vi "Eraser.vi"(8 "error in (no error)":errorcluster, 9 "point(x,y)":cluster{"x":i16, "y":i16}, 10 "Radio Buttons":T8=enum."Ellipse", 11 "Data in":T1={"Class"={"Ants"=refnum, "Layer"=refnum, "Templates"=refnum, "Icon"=refnum, "Glyph"=refnum, "Settings"=refnum, "Tools"=refnum}, "Ref"={"Add Layer"=refnum, "Remove Layer"=refnum, "Line Text"=[], "Body Text Spec"=refnum, "DNL_Font"=refnum, "glyph path str"=refnum, "templates path str"=refnum, "Arrow Up"=refnum, "Arrow Down"=refnum, "IE VI Ref"=refnum, "Glyphs tree"=refnum, "Templates tree"=refnum, "Layer Icon Text"=refnum, "Layer Template"=refnum, "Body Text"=refnum, "Search Templates"=refnum, "TextMarker"=refnum, "Tab Control"=refnum, "Search Glyphs"=refnum, "Line Color"=refnum, "DNL_Glyphs []"=refnum, "Fill Color"=refnum, "Tools"=refnum, "Icon"=refnum, "Preview"=refnum, "Ants"=refnum, "Terminals"=refnum, "menu reference"=refnum, "LayerNames"=[], "GlyphLoadAnimation"=refnum, "TemplateLoadAnimation"=refnum, "refreshGlyphs"=refnum, "refreshTemplates"=refnum}, "Support"={"AntsRect"={"left"=0, "top"=0, "right"=0, "bottom"=0}, "Mouse Move Coords"={"Horizontal"=0, "Vertical"=0}, "Mouse Down Coords"={"Horizontal"=0, "Vertical"=0}, "Temp Coord"={"Horizontal"=0, "Vertical"=0}, "Action"=enum."Default", "Edge Color"=4914962, "Fill Color"=16860, "Mouse Down?"=FALSE, "Draft Mode?"=FALSE, "Temp Icon"=bytes[3102], "CTRL Pressed"=FALSE, "Move Selection?"=FALSE, "AntsRect Orig"={"left"=0, "top"=0, "right"=0, "bottom"=0}, "Text"="", "TM Set?"=FALSE, "Mouse inside icon?"=FALSE, "Tool (old value)"=0, "Pencil Move Color"=0, "Swap Colors?"=FALSE, "Shift pressed?"=FALSE}}) -> (0 "error out":errorcluster, 3 "Data out":T1={"Class"={"Ants"=refnum, "Layer"=refnum, "Templates"=refnum, "Icon"=refnum, "Glyph"=refnum, "Settings"=refnum, "Tools"=refnum}, "Ref"={"Add Layer"=refnum, "Remove Layer"=refnum, "Line Text"=[], "Body Text Spec"=refnum, "DNL_Font"=refnum, "glyph path str"=refnum, "templates path str"=refnum, "Arrow Up"=refnum, "Arrow Down"=refnum, "IE VI Ref"=refnum, "Glyphs tree"=refnum, "Templates tree"=refnum, "Layer Icon Text"=refnum, "Layer Template"=refnum, "Body Text"=refnum, "Search Templates"=refnum, "TextMarker"=refnum, "Tab Control"=refnum, "Search Glyphs"=refnum, "Line Color"=refnum, "DNL_Glyphs []"=refnum, "Fill Color"=refnum, "Tools"=refnum, "Icon"=refnum, "Preview"=refnum, "Ants"=refnum, "Terminals"=refnum, "menu reference"=refnum, "LayerNames"=[], "GlyphLoadAnimation"=refnum, "TemplateLoadAnimation"=refnum, "refreshGlyphs"=refnum, "refreshTemplates"=refnum}, "Support"={"AntsRect"={"left"=0, "top"=0, "right"=0, "bottom"=0}, "Mouse Move Coords"={"Horizontal"=0, "Vertical"=0}, "Mouse Down Coords"={"Horizontal"=0, "Vertical"=0}, "Temp Coord"={"Horizontal"=0, "Vertical"=0}, "Action"=enum."Default", "Edge Color"=4914962, "Fill Color"=16860, "Mouse Down?"=FALSE, "Draft Mode?"=FALSE, "Temp Icon"=bytes[3102], "CTRL Pressed"=FALSE, "Move Selection?"=FALSE, "AntsRect Orig"={"left"=0, "top"=0, "right"=0, "bottom"=0}, "Text"="", "TM Set?"=FALSE, "Mouse inside icon?"=FALSE, "Tool (old value)"=0, "Pencil Move Color"=0, "Swap Colors?"=FALSE, "Shift pressed?"=FALSE}})   [LabVIEW 2021, in "Tools Paint.lvclass"]
uses:
  <resource>/plugins/NIIconEditor/Class/Tools/Tools Paint.lvclass
  <resource>/plugins/NIIconEditor/Controls/Tools.ctl
  <resource>/plugins/NIIconEditor/Controls/Pen.ctl
  <resource>/plugins/NIIconEditor/Controls/Line.ctl
  <resource>/plugins/NIIconEditor/Controls/Dropper.ctl
  <resource>/plugins/NIIconEditor/Controls/Fill.ctl
  <resource>/plugins/NIIconEditor/Controls/IERect.ctl
  <resource>/plugins/NIIconEditor/Controls/FRect.ctl
  <resource>/plugins/NIIconEditor/Controls/Circle.ctl
  <resource>/plugins/NIIconEditor/Controls/FCircle.ctl
  <resource>/plugins/NIIconEditor/Controls/Rubber.ctl
  <resource>/plugins/NIIconEditor/Controls/Text.ctl
  <resource>/plugins/NIIconEditor/Controls/Selection.ctl
  <resource>/plugins/NIIconEditor/Controls/Move.ctl
  <resource>/plugins/NIIconEditor/Controls/Global Data.ctl
  <resource>/plugins/NIIconEditor/Class/Ants/Ants.lvclass
  <resource>/plugins/NIIconEditor/Class/FakedArray/FakedArray.lvclass
  <vilib>/LabVIEW Icon API/lv_icon/Classes/Icon/Icon.lvclass
  <resource>/plugins/NIIconEditor/Class/Icon Library/Glyph.lvclass
  <resource>/plugins/NIIconEditor/Class/Settings/Settings.lvclass
  <resource>/plugins/NIIconEditor/Controls/IE Classes.ctl
  <resource>/plugins/NIIconEditor/Controls/References Cluster.ctl
  <resource>/plugins/NIIconEditor/Controls/SupportClass.ctl
  <vilib>/Utility/miscctls.llb/LVPoint32TypeDef.ctl
  <resource>/plugins/NIIconEditor/Controls/SupportClass_Action.ctl
  <vilib>/LabVIEW Icon API/lv_icon/Controls/IEColor.ctl
  <vilib>/LabVIEW Icon API/lv_icon/Classes/Icon Framework/Icon Framework.lvclass
  C:/Users/J63553/Projects/_LabVIEW Community/labview-icon-editor/vi.lib/LabVIEW Icon API/lv_icon/Classes/Layer/Layer.lvclass
  <vilib>/LabVIEW Icon API/lv_icon/lv_icon.lvlib
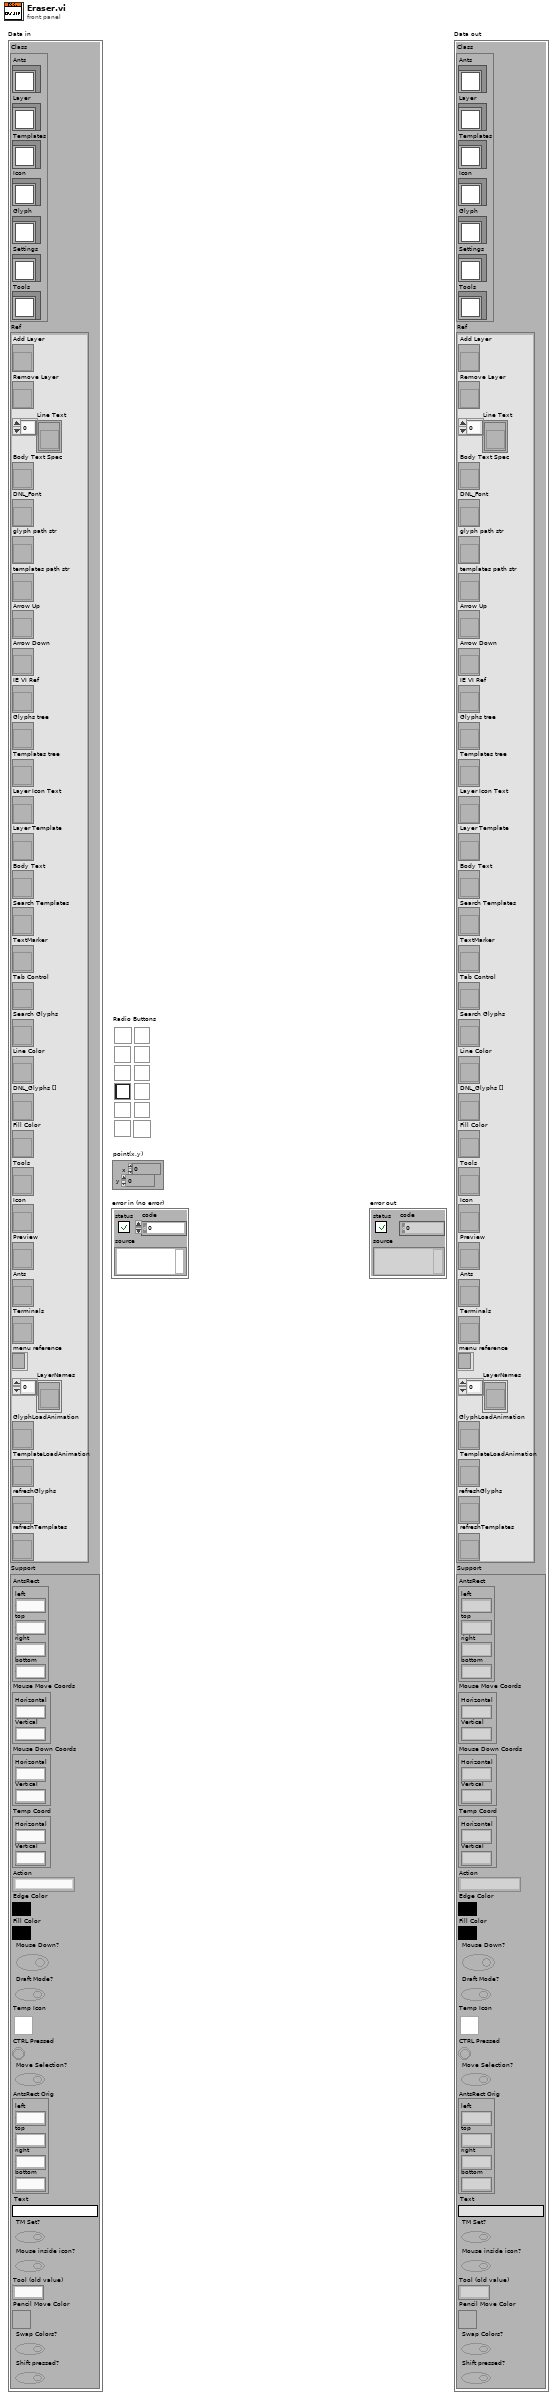
[diagram p1: front panel]
types:
  T1 = typedef "lv_icon.lvlib/Global Data.ctl" = cluster{"Class":T2, "Ref":T3, "Support":T4}
  T2 = typedef "IE Classes.ctl" = cluster{"Ants":refnum<class "Ants.lvclass">, "Layer":refnum<class "FakedArray.lvclass">, "Templates":refnum<class "FakedArray.lvclass">, "Icon":refnum<class "Icon.lvclass">, "Glyph":refnum<class "Glyph.lvclass">, "Settings":refnum<class "Settings.lvclass">, "Tools":refnum<class "Tools Paint.lvclass">}
  T3 = typedef "lv_icon.lvlib/References Cluster.ctl" = cluster{"Add Layer":refnum<vi>, "Remove Layer":refnum<vi>, "Line Text":refnum<vi>[], "Body Text Spec":refnum<vi>, "DNL_Font":refnum<vi>, "glyph path str":refnum<vi>, "templates path str":refnum<vi>, "Arrow Up":refnum<vi>, "Arrow Down":refnum<vi>, "IE VI Ref":refnum<vi>, "Glyphs tree":refnum<vi>, "Templates tree":refnum<vi>, "Layer Icon Text":refnum<vi>, "Layer Template":refnum<vi>, "Body Text":refnum<vi>, "Search Templates":refnum<vi>, "TextMarker":refnum<vi>, "Tab Control":refnum<vi>, "Search Glyphs":refnum<vi>, "Line Color":refnum<vi>, "DNL_Glyphs []":refnum<vi>, "Fill Color":refnum<vi>, "Tools":refnum<vi>, "Icon":refnum<vi>, "Preview":refnum<vi>, "Ants":refnum<vi>, "Terminals":refnum<vi>, "menu reference":refnum<k9>, "LayerNames":refnum<vi>[], "GlyphLoadAnimation":refnum<vi>, "TemplateLoadAnimation":refnum<vi>, "refreshGlyphs":refnum<vi>, "refreshTemplates":refnum<vi>}
  T4 = typedef "SupportClass.ctl" = cluster{"AntsRect":cluster{"left":i16, "top":i16, "right":i16, "bottom":i16}, "Mouse Move Coords":T5, "Mouse Down Coords":T5, "Temp Coord":T5, "Action":T6, "Edge Color":T7, "Fill Color":T7, "Mouse Down?":bool, "Draft Mode?":bool, "Temp Icon":picture, "CTRL Pressed":bool, "Move Selection?":bool, "AntsRect Orig":cluster{"left":i16, "top":i16, "right":i16, "bottom":i16}, "Text":string, "TM Set?":bool, "Mouse inside icon?":bool, "Tool (old value)":u32, "Pencil Move Color":u32, "Swap Colors?":bool, "Shift pressed?":bool}
  T5 = typedef "LVPoint32TypeDef.ctl" = cluster{"Horizontal":i32, "Vertical":i32}
  T6 = typedef "SupportClass_Action.ctl" = enum16{"Default", "Move Selection", "Glyph Library", "Tool"}
  T7 = typedef "IEColor.ctl" = u32
  T8 = typedef "Tools.ctl" = enum32{"Pencil", "Line", "Dropper", "Fill", "Rectangle", "Filled Rectangle", "Ellipse", "Filled Ellipse", "Eraser", "Text", "Select", "Move"}
  T9 = typedef "lv_icon.lvlib/INI Data.ctl" = cluster{"Show Terminals?":bool, "Text":cluster{"Font":T10, "Alignment":T11, "Size":T12}, "3rd party Templates":cluster{"Store 3rd party Templates?":bool, "Folder Name":string}, "Merge user layers on commit":bool, "Body Text":T13, "Fill Color":T7, "Edge Color":T7, "Tab":u16, "Tool":T8, "Disable Layers?":bool}
  T10 = typedef "Font.ctl" = string
  T11 = typedef "Alignment.ctl" = u16
  T12 = typedef "Font Size.ctl" = u8
  T13 = typedef "BodyText.ctl" = cluster{"Line 1 text":string, "Line 2 text":string, "Line 3 text":string, "Line 4 text":string, "Line 1 color":u32, "Line 2 color":u32, "Line 3 color":u32, "Line 4 color":u32, "Body Text Spec":cluster{"Font":T10, "Alignment":T11, "Size":u8}, "Center text vertically":bool, "Capitalize Text":bool}
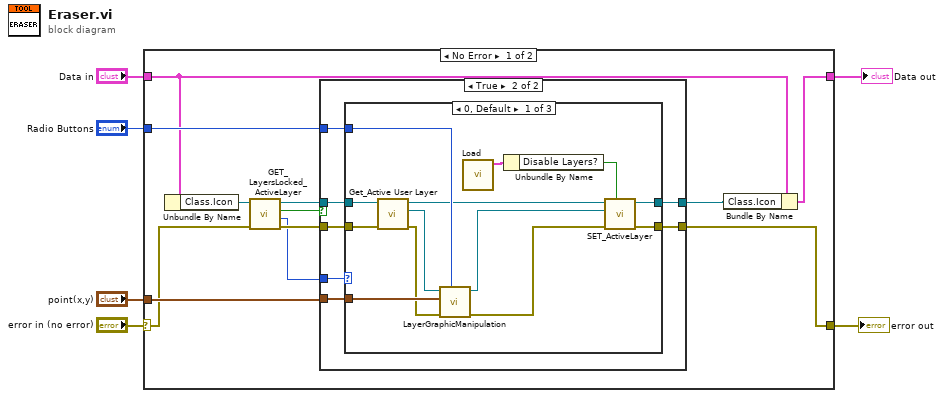
[diagram p0: block diagram]
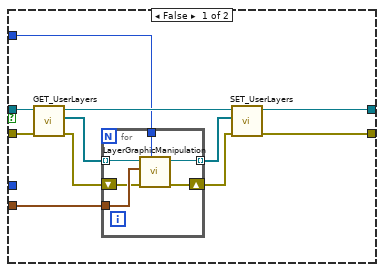
[diagram p2: hidden frame]
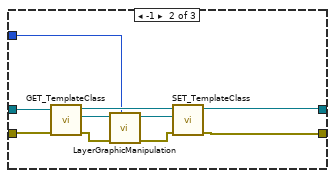
[diagram p3: hidden frame]
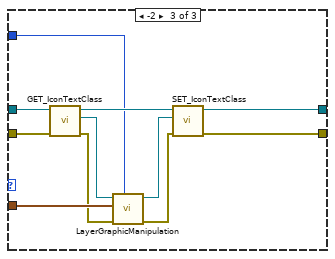
[diagram p4: hidden frame]
diagram:
  n1 = case shown="No Error" "error in (no error)" {
    selector: "error in (no error)" -> [w11 w78]
    tunnel: [w8 w78] -> w5
    tunnel: "point(x,y)" -> [w18 _]
    tunnel: "Radio Buttons" -> [w17 _]
    tunnel: "Data in" -> [w10 w77]
    tunnel: [w7 w77] -> w1
    frame No Error {
      n2 = Unbundle By Name(w10) -> ("Class.Icon"=w12:refnum<class "Icon.lvclass">)
      n3 = call-dynamic "GET_LayersLocked_ActiveLayer.vi"("error in (no error)"=w11, "Icon.lvclass in"=w12) -> ("error out"=w15:errorcluster, "Active Layer"=w13:i32, "Layers Locked?"=w14:bool, "Icon.lvclass out"=w16:refnum<class "Icon.lvclass">)  [unwired: 6 out]
      n4 = case shown="True" w14 {
        tunnel: w18 -> [w24 w39]
        tunnel: w17 -> [w23 w38]
        tunnel: [w21 w37] -> w9
        tunnel: [w19 w36] -> w8
        tunnel: w16 -> [w22 w41]
        tunnel: w15 -> [w20 w40]
        tunnel: w13 -> [_ w42]
        frame False {
          n5 = call-dynamic "GET_UserLayers.vi"("error in (no error)"=w20, "Icon.lvclass in"=w22) -> ("error out"=w29:errorcluster, "All Layers"=w28:refnum<class "Layer.lvclass">[], "Icon.lvclass out"=w26:refnum<class "Icon.lvclass">)  [unwired: 7 out]
          n6 = for {
            tunnel: w28 -> [w34] mode=indexing
            tunnel: w24 -> [w35]
            tunnel: [w32] -> w27 mode=indexing
            shift-right: [w31] -> w25
            shift-left: w29 -> [w33]
            tunnel: w23 -> [w30]
            n7 = call <resource>:"LayerGraphicManipulation.vi"("Radio Buttons"=w30, "error in"=w33, "point(x,y)"=w35, "Layer.lvclass"=w34) -> ("error out"=w31:errorcluster, "Layer.lvclass out"=w32:refnum<class "Layer.lvclass">)  [unwired: 2 in, 4 out]
          }
          n8 = call-dynamic "SET_UserLayers.vi"("error in (no error)"=w25, "Layers"=w27, "Icon.lvclass in"=w26) -> ("error out"=w19:errorcluster, "Icon.lvclass out"=w21:refnum<class "Icon.lvclass">)  [unwired: 7 out]
        }
        frame True {
          n9 = case shown="0, Default" w42 {
            tunnel: w41 -> [w55 w65 w76]
            tunnel: w40 -> [w54 w63 w75]
            tunnel: w39 -> [w52 _ w73]
            tunnel: w38 -> [w51 w56 w66]
            tunnel: [w48 w58 w68] -> w37
            tunnel: [w46 w57 w67] -> w36
            frame 0, Default {
              n10 = call-dynamic "Get_Active User Layer.vi"("error in (no error)"=w54, "Icon in"=w55) -> ("error out"=w49:errorcluster, "Layer.lvclass"=w53:refnum<class "Layer.lvclass">, "Icon out"=w50:refnum<class "Icon.lvclass">)  [unwired: 7 out]
              n11 = call <resource>:"LayerGraphicManipulation.vi"("Radio Buttons"=w51, "error in"=w49, "point(x,y)"=w52, "Layer.lvclass"=w53) -> ("error out"=w47:errorcluster, "Layer.lvclass out"=w45:refnum<class "Layer.lvclass">)  [unwired: 2 in, 4 out]
              n12 = call <resource>:"Load.vi"() -> ("INI Data"=w44:T9)  [unwired: 3 in, 8 out]
              n13 = Unbundle By Name(w44) -> ("Disable Layers?"=w43:bool)
              n14 = call-dynamic "SET_ActiveLayer.vi"("Combine User Layers?"=w43, "error in (no error)"=w47, "Layer.lvclass"=w45, "Icon.lvclass in"=w50) -> ("error out"=w46:errorcluster, "Icon.lvclass out"=w48:refnum<class "Icon.lvclass">)  [unwired: 6 out]
            }
            frame -1 {
              n15 = call-dynamic "GET_TemplateClass.vi"("error in (no error)"=w63, "Icon.lvclass in"=w65) -> ("error out"=w62:errorcluster, "Icon Framework.lvclass"=w64:refnum<class "Icon Framework.lvclass">, "Icon.lvclass out"=w61:refnum<class "Icon.lvclass">)  [unwired: 7 out]
              n16 = call <resource>:"LayerGraphicManipulation.vi"("Radio Buttons"=w56, "error in"=w62, "Layer.lvclass"=w64) -> ("error out"=w59:errorcluster, "Layer.lvclass out"=w60:refnum<class "Icon Framework.lvclass">)  [unwired: 3 in, 4 out]
              n17 = call-dynamic "SET_TemplateClass.vi"("error in (no error)"=w59, "Icon Framework.lvclass"=w60, "Icon.lvclass in"=w61) -> ("error out"=w57:errorcluster, "Icon.lvclass out"=w58:refnum<class "Icon.lvclass">)  [unwired: 7 out]
            }
            frame -2 {
              n18 = call-dynamic "GET_IconTextClass.vi"("error in (no error)"=w75, "Icon.lvclass in"=w76) -> ("error out"=w72:errorcluster, "Icon Framework.lvclass"=w74:refnum<class "Icon Framework.lvclass">, "Icon.lvclass out"=w71:refnum<class "Icon.lvclass">)  [unwired: 7 out]
              n19 = call <resource>:"LayerGraphicManipulation.vi"("Radio Buttons"=w66, "error in"=w72, "point(x,y)"=w73, "Layer.lvclass"=w74) -> ("error out"=w69:errorcluster, "Layer.lvclass out"=w70:refnum<class "Icon Framework.lvclass">)  [unwired: 2 in, 4 out]
              n20 = call-dynamic "SET_IconTextClass.vi"("error in (no error)"=w69, "Icon Framework.lvclass"=w70, "Icon.lvclass in"=w71) -> ("error out"=w67:errorcluster, "Icon.lvclass out"=w68:refnum<class "Icon.lvclass">)  [unwired: 7 out]
            }
          }
        }
      }
      n21 = Bundle By Name(cluster=w10, "Class.Icon"=w9) -> (w7:T1)
    }
    frame Error {
    }
  }
  "error out" <- w5
  "Data out" <- w1
